vi "Status Monitor - Reader - Graphical User Interface.vi"() -> ()   [LabVIEW 2017, in "Status Monitor Library.lvlib"]
doc: "Graphical user interface, used to monitor status from several units on a network."
uses:
  Status Monitor Library.lvlib
  Communications/Typedefs/DTACQ Module Carrier Status.ctl
  Communications/Typedefs/DTACQ Status--Enum.ctl
  Communications/Communications Library.lvlib
panel:
  in  "Cancel Button":bool
  out "URL":string
  out "Shared Variable Name":string
  out "Demuxing":bool
  out "Total Samples":i32
  out "Post-Buffered Samples":i32
  out "Pre-Buffered Samples":i32
  out "Device State":T1(ring)
  in  "Module Carrier":i32
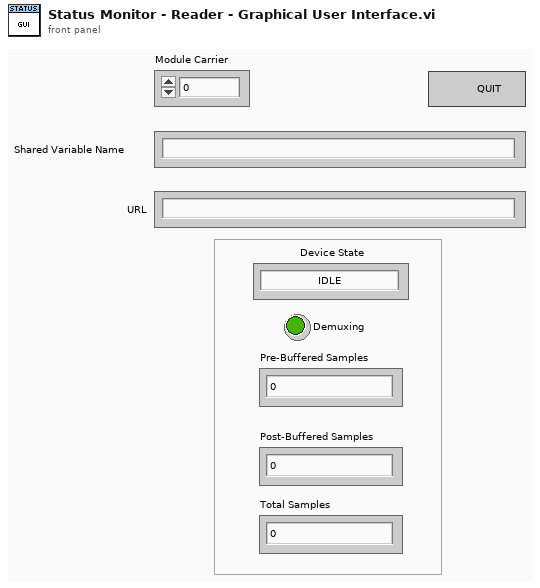
[diagram p1: front panel]
types:
  T1 = enum16{"IDLE", "ARM", "RUN_PRE-TRIGGER", "RUN_POST-TRIGGER", "POST_PROCESS", "CLEANUP"}
  T2 = typedef "Shared Variables Library.lvlib/Share Variable and Description--Cluster.ctl" = cluster{"Shared Variable Reference":refnum<k21>, "Shared Variable Description":T3}
  T3 = typedef "Shared Variables Library.lvlib/Shared Variable Properties--Cluster.ctl" = cluster{"Name":string, "URL":string, "Data Type":variant}
  T4 = typedef "Communications Library.lvlib/DTACQ Module Carrier Status.ctl" = cluster{"DTACQ State":T5, "Pre-Trigger Samples":i32, "Post-Trigger Samples":i32, "Total Samples":i32, "Post Processing":bool}
  T5 = typedef "Communications Library.lvlib/DTACQ Status--Enum.ctl" = enum16{"IDLE", "ARM", "RUN_PRE-TRIGGER", "RUN_POST-TRIGGER", "POST_PROCESS", "CLEANUP"}
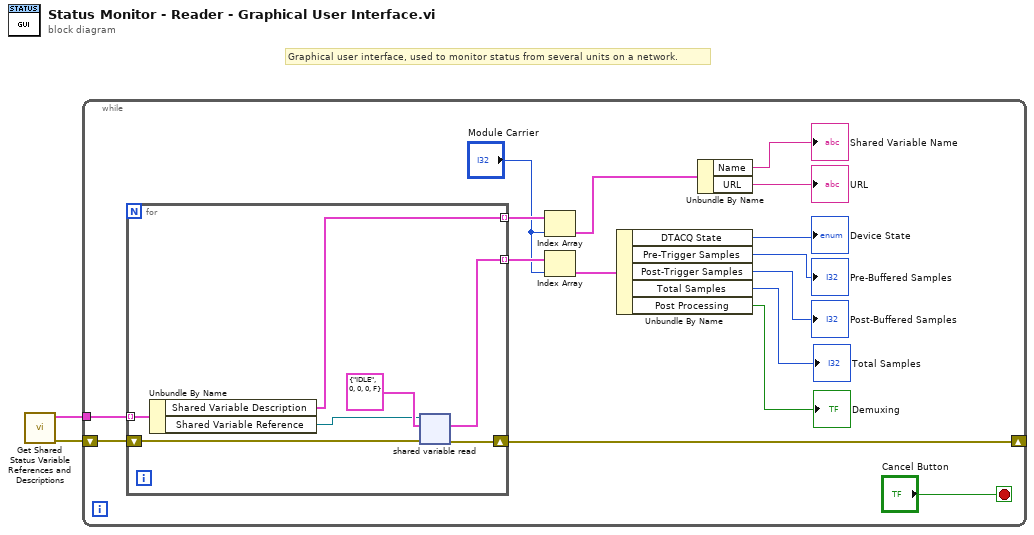
[diagram p0: block diagram]
diagram:
  # "Graphical user interface, used to monitor status from several units on a network."
  n1 = call "Get Shared Status Variable References and Descriptions.vi"() -> ("error out"=w2:errorcluster, "Shared Variables and Descriptions"=w1:T2[])  [unwired: 10 in]
  n2 = while {
    tunnel: w1 -> [w17]
    shift-right: [w4] -> _
    shift-left: w2 -> [w18]
    stop <- "Cancel Button" stop-if-true
    n3 = for {
      tunnel: w17 -> [w20] mode=indexing
      tunnel: [w21] -> w16 mode=indexing
      tunnel: [w19] -> w15 mode=indexing
      shift-right: [w22] -> w4
      shift-left: w18 -> [w25]
      n4 = Unbundle By Name(w20) -> ("Shared Variable Description"=w19:T3, "Shared Variable Reference"=w23:refnum<k21>)
      n5 = shared-variable-read(w23, w25, T4 {"DTACQ State"=enum."IDLE", "Pre-Trigger Samples"=0, "Post-Trigger Samples"=0, "Total Samples"=0, "Post Processing"=FALSE} ("Module Carrier Status")) -> (w22:errorcluster, w21:T4)  [unwired: 2 out]
    }
    n6 = Index Array(array=w15, index="Module Carrier") -> (element=w13:T3)
    n7 = Index Array(array=w16, index="Module Carrier") -> (element=w12:T4)
    n8 = Unbundle By Name(w12) -> ("DTACQ State"=→"Device State":T5, "Pre-Trigger Samples"=→"Pre-Buffered Samples":i32, "Post-Trigger Samples"=→"Post-Buffered Samples":i32, "Total Samples"=→"Total Samples":i32, "Post Processing"=→"Demuxing":bool)
    n9 = Unbundle By Name(w13) -> ("Name"=→"Shared Variable Name":string, "URL"=→"URL":string)
  }
